vi "Register gRPC Messages.vi"(8 "error in (no error)":errorcluster, 11 "gRPC ID":T1) -> (0 "error out":errorcluster, 3 "gRPC ID Out":T1)   [LabVIEW 2020, in "Session Management Client_v1.lvlib"]
uses:
  Session Management Client_v1.lvlib
  <vilib>/gRPC/LabVIEW gRPC Library/Shared/grpcId.ctl
  <vilib>/gRPC/LabVIEW gRPC Library/Server API/typeDefs/Message Metadata.ctl
  <vilib>/gRPC/LabVIEW gRPC Library/Server API/typeDefs/Message Element Metadata.ctl
  <vilib>/gRPC/LabVIEW gRPC Library/Server API/typeDefs/Message Element Type.ctl
  <vilib>/gRPC/LabVIEW gRPC Library/grpc-lvsupport-release.lvlib
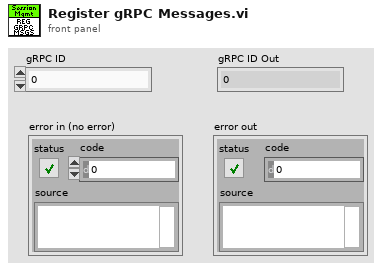
[diagram p1: front panel]
types:
  T1 = typedef "grpc-lvsupport-release.lvlib/grpcId.ctl" = u64
  T2 = typedef "grpc-lvsupport-release.lvlib/Message Metadata.ctl" = cluster{"Version":i32, "Name":string, "Type Url":string, "Elements":T3[]}
  T3 = typedef "grpc-lvsupport-release.lvlib/Message Element Metadata.ctl" = cluster{"Embedded Message Name":string, "Protobuf Index":i32, "MessageElementType":T4, "Repeated":bool}
  T4 = typedef "grpc-lvsupport-release.lvlib/Message Element Type.ctl" = enum32{"Int32Value", "FloatValue", "DoubleValue", "BoolValue", "StringValue", "MessageValue", "Int64Value", "UInt32Value", "UInt64Value", "EnumValue", "Bytes", "Fixed64", "Fixed32", "SFixed64", "SFixed32", "SInt64", "SInt32"}
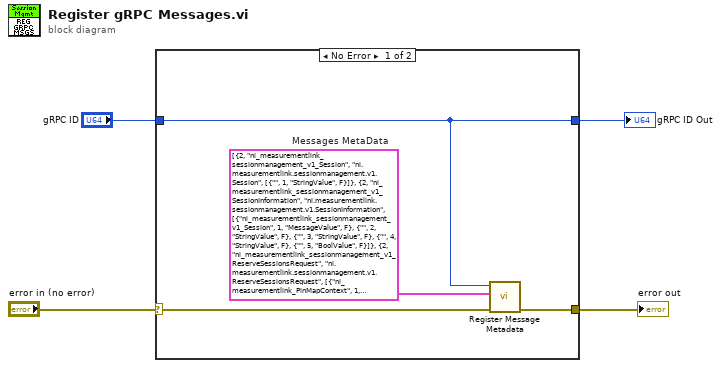
[diagram p0: block diagram]
diagram:
  n1 = case shown="No Error" "error in (no error)" {
    selector: "error in (no error)" -> [w6 w10]
    tunnel: [w5 w9] -> w1
    tunnel: [w8 w10] -> w4
    tunnel: "gRPC ID" -> [w5 w9]
    frame No Error {
      w7 = T2[] [{"Version"=2, "Name"="ni_measurementlink_sessionmanagement_v1_Session", "Type Url"="ni.measurementlink.sessionmanagement.v1.Session", "Elements"=[{"Embedded Message Name"="", "Protobuf Index"=1, "MessageElementType"=enum."StringValue", "Repeated"=FALSE}]}, {"Version"=2, "Name"="ni_measurementlink_sessionmanagement_v1_SessionInformation", "Type Url"="ni.measurementlink.sessionmanagement.v1.SessionInformation", "Elements"=[{"Embedded Message Name"="ni_measurementlink_sessionmanagement_v1_Session", "Protobuf Index"=1, "MessageElementType"=enum."MessageValue", "Repeated"=FALSE}, {"Embedded Message Name"="", "Protobuf Index"=2, "MessageElementType"=enum."StringValue", "Repeated"=FALSE}, {"Embedded Message Name"="", "Protobuf Index"=3, "MessageElementType"=enum."StringValue", "Repeated"=FALSE}, {"Embedded Message Name"="", "Protobuf Index"=4, "MessageElementType"=enum."StringValue", "Repeated"=FALSE}, {"Embedded Message Name"="", "Protobuf Index"=5, "MessageElementType"=enum."BoolValue", "Repeated"=FALSE}]}, {"Version"=2, "Name"="ni_measurementlink_sessionmanagement_v1_ReserveSessionsRequest", "Type Url"="ni.measurementlink.sessionmanagement.v1.ReserveSessionsRequest", "Elements"=[{"Embedded Message Name"="ni_measurementlink_PinMapContext", "Protobuf Index"=1, "MessageElementType"=enum."MessageValue", "Repeated"=FALSE}, {"Embedded Message Name"="", "Protobuf Index"=2, "MessageElementType"=enum."StringValue", "Repeated"=TRUE}, {"Embedded Message Name"="", "Protobuf Index"=3, "MessageElementType"=enum."StringValue", "Repeated"=FALSE}, {"Embedded Message Name"="", "Protobuf Index"=4, "MessageElementType"=enum."Int32Value", "Repeated"=FALSE}]}, {"Version"=2, "Name"="ni_measurementlink_sessionmanagement_v1_ReserveSessionsResponse", "Type Url"="ni.measurementlink.sessionmanagement.v1.ReserveSessionsResponse", "Elements"=[{"Embedded Message Name"="ni_measurementlink_sessionmanagement_v1_SessionInformation", "Protobuf Index"=1, "MessageElementType"=enum."MessageValue", "Repeated"=TRUE}]}, {"Version"=2, "Name"="ni_measurementlink_sessionmanagement_v1_UnreserveSessionsRequest", "Type Url"="ni.measurementlink.sessionmanagement.v1.UnreserveSessionsRequest", "Elements"=[{"Embedded Message Name"="ni_measurementlink_sessionmanagement_v1_SessionInformation", "Protobuf Index"=1, "MessageElementType"=enum."MessageValue", "Repeated"=TRUE}]}, {"Version"=2, "Name"="ni_measurementlink_sessionmanagement_v1_UnreserveSessionsResponse", "Type Url"="ni.measurementlink.sessionmanagement.v1.UnreserveSessionsResponse", "Elements"=[]}, {"Version"=2, "Name"="ni_measurementlink_sessionmanagement_v1_RegisterSessionsRequest", "Type Url"="ni.measurementlink.sessionmanagement.v1.RegisterSessionsRequest", "Elements"=[{"Embedded Message Name"="ni_measurementlink_sessionmanagement_v1_SessionInformation", "Protobuf Index"=1, "MessageElementType"=enum."MessageValue", "Repeated"=TRUE}]}, {"Version"=2, "Name"="ni_measurementlink_sessionmanagement_v1_RegisterSessionsResponse", "Type Url"="ni.measurementlink.sessionmanagement.v1.RegisterSessionsResponse", "Elements"=[]}, {"Version"=2, "Name"="ni_measurementlink_sessionmanagement_v1_UnregisterSessionsRequest", "Type Url"="ni.measurementlink.sessionmanagement.v1.UnregisterSessionsRequest", "Elements"=[{"Embedded Message Name"="ni_measurementlink_sessionmanagement_v1_SessionInformation", "Protobuf Index"=1, "MessageElementType"=enum."MessageValue", "Repeated"=TRUE}]}, {"Version"=2, "Name"="ni_measurementlink_sessionmanagement_v1_UnregisterSessionsResponse", "Type Url"="ni.measurementlink.sessionmanagement.v1.UnregisterSessionsResponse", "Elements"=[]}, {"Version"=2, "Name"="ni_measurementlink_sessionmanagement_v1_ReserveAllRegisteredSessionsRequest", "Type Url"="ni.measurementlink.sessionmanagement.v1.ReserveAllRegisteredSessionsRequest", "Elements"=[{"Embedded Message Name"="", "Protobuf Index"=1, "MessageElementType"=enum."Int32Value", "Repeated"=FALSE}]}, {"Version"=2, "Name"="ni_measurementlink_sessionmanagement_v1_ReserveAllRegisteredSessionsResponse", "Type Url"="ni.measurementlink.sessionmanagement.v1.ReserveAllRegisteredSessionsResponse", "Elements"=[{"Embedded Message Name"="ni_measurementlink_sessionmanagement_v1_SessionInformation", "Protobuf Index"=1, "MessageElementType"=enum."MessageValue", "Repeated"=TRUE}]}, {"Version"=2, "Name"="ni_measurementlink_PinMapContext", "Type Url"="ni.measurementlink.PinMapContext", "Elements"=[{"Embedded Message Name"="", "Protobuf Index"=1, "MessageElementType"=enum."StringValue", "Repeated"=FALSE}, {"Embedded Message Name"="", "Protobuf Index"=2, "MessageElementType"=enum."Int32Value", "Repeated"=TRUE}]}]  # Messages MetaData
      n2 = call <vilib>:"Register Message Metadata.vi"("error in"=w6, "Messages"=w7, "gRPCid in"=w5) -> ("error out"=w8:errorcluster)  [unwired: 7 in, 1 out]
    }
    frame Error {
    }
  }
  "error out" <- w4
  "gRPC ID Out" <- w1
